vi "test_cmd.vi"() -> ()   [LabVIEW 2017]
panel:
  out "standard error":string caption="표준 에러"
  out "standard output":string caption="표준 출력"
  in  "command line":string caption="명령 라인"
  # "netstat"
  # "pwd"
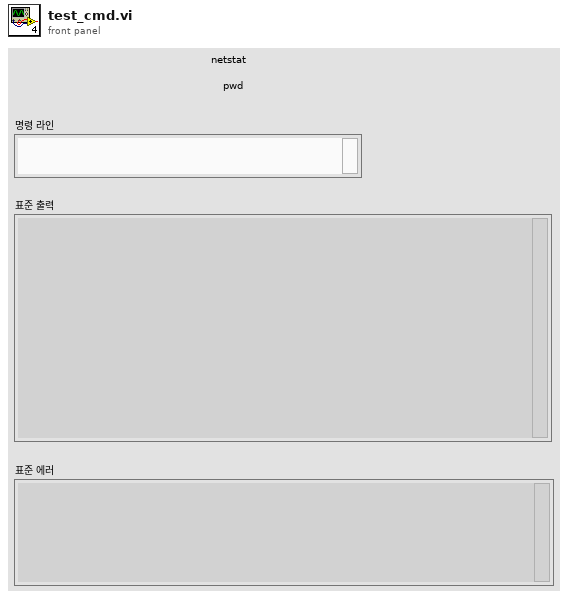
[diagram p1: front panel]
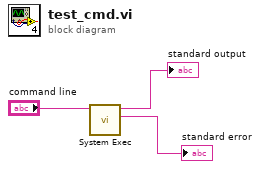
[diagram p0: block diagram]
diagram:
  n1 = call <vilib>:"System Exec.vi"("command line"="command line") -> ("standard error"=→"standard error":string, "standard output"=→"standard output":string)  [unwired: 7 in, 2 out]
